vi "Map Poly to Pixels.vi"(9 "Draw Area Size":T1, 10 "Position":cluster{"Left":dbl, "Top":dbl}, 11 "Coords":cluster{"Horizontal":dbl, "Vertical":dbl}[](array[cluster])) -> (3 "Coords":cluster{"Horizontal":dbl, "Vertical":dbl}[](array[cluster]))   [LabVIEW 2025]
uses:
  <vilib>/Utility/miscctls.llb/LVBoundsTypeDef.ctl
  Global Settings.vi
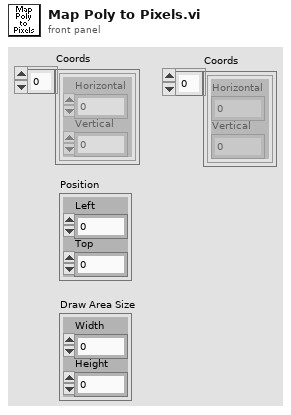
[diagram p1: front panel]
types:
  T1 = typedef "LVBoundsTypeDef.ctl" = cluster{"Width":u32, "Height":u32}
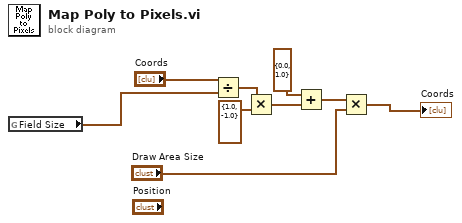
[diagram p0: block diagram]
diagram:
  n1 = global read "Global Settings.vi" "Field Size"() -> (w1:cluster{"width":dbl, "height":dbl})
  n2 = Divide(x="Coords", y=w1) -> (x/y=w5:cluster{dbl, dbl}[])
  n3 = Multiply(x=w5, y=cluster{"Width":dbl, "Height":dbl} {"Width"=1.0, "Height"=-1.0} ("Bounds")) -> (x*y=w4:cluster{dbl, dbl}[])
  n4 = Add(x=cluster{"Width":dbl, "Height":dbl} {"Width"=0.0, "Height"=1.0} ("Bounds"), y=w4) -> (x+y=w3:cluster{dbl, dbl}[])
  n5 = Multiply(x=w3, y="Draw Area Size") -> (x*y=→"Coords":cluster{dbl, dbl}[])
